vi "postPubDataUE.vi"(6 "newValue (T)":bool=TRUE, 8 "error in (no error)":errorcluster, 9 "value":variant, 10 "pubDataSV":T1=enum."LoopTime_ms", 11 "Model in":refnum<class "Model.lvclass">) -> (0 "error out":errorcluster, 3 "Model out":refnum<class "Model.lvclass">)   [LabVIEW 2016, in "Model.lvclass"]
doc: "Updates the variable value."
uses:
  Model.lvclass
  Typedefs/PubDataSV.ctl
  Model.lvclass/Model.ctl
  PubSubDataEvent/PubSubDataEvent.lvclass/PubSubDataEvent.ctl
  Typedefs/StateValue.ctl
  Typedefs/RejectedCommand.ctl
  Typedefs/CommandValue.ctl
  ComponentTemplateCore/ComponentModel/ComponentModel/Typedefs/ComponentStateValues.ctl
  PubSubDataEvent/PubSubDataEvent.lvclass
  Typedefs/EXATypedefs.lvlib
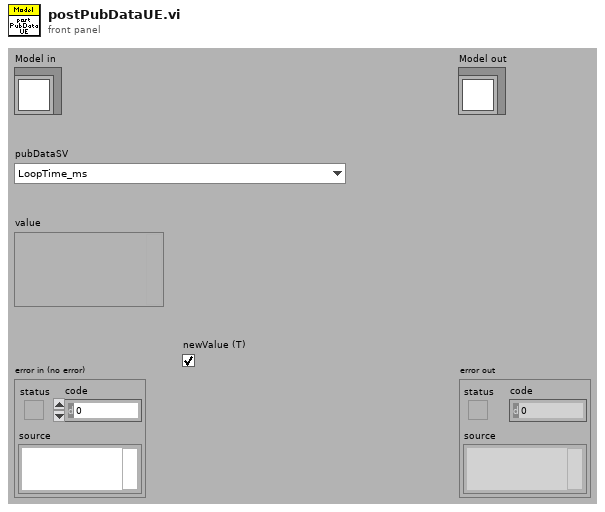
[diagram p1: front panel]
types:
  T1 = typedef "EXATypedefs.lvlib/PubDataSV.ctl" = enum16{"DetailedState", "ErrorCode", "Heartbeat", "LoopTime_ms", "LoopTimeOutOfRange", "RejectedCommand", "SummaryState", "Timestamp"}
  T2 = typedef "EXATypedefs.lvlib/PubDataEvents.ctl" = cluster{"DetailedState":refnum<user-event>, "ErrorCode":refnum<user-event>, "Heartbeat":refnum<user-event>, "LoopTime_ms":refnum<user-event>, "LoopTimeOutOfRange":refnum<user-event>, "RejectedCommand":refnum<user-event>, "SummaryState":refnum<user-event>, "Timestamp":refnum<user-event>, "AppliedSettingsMatchStart":refnum<user-event>, "SettingsApplied":refnum<user-event>, "SettingVersions":refnum<user-event>}
  T3 = typedef "EXATypedefs.lvlib/StateValue.ctl" = enum16{"DisabledState", "EnabledState", "FaultState", "OffState", "StandbyState"}
  T4 = typedef "EXATypedefs.lvlib/RejectedCommand.ctl" = cluster{"CommandValue":T5, "StateValue":T3, "Time Stamp":dbl}
  T5 = typedef "EXATypedefs.lvlib/CommandValue.ctl" = enum16{"ClearError", "Disable", "Enable", "Exit", "GoToStandby", "OnHeartbeat", "OnIncomingMessagingError", "OnInterrupt", "Start"}
  T6 = typedef "ComponentStateValues.ctl" = enum16{"Off", "Standby", "Enabled", "Disabled", "Fault"}
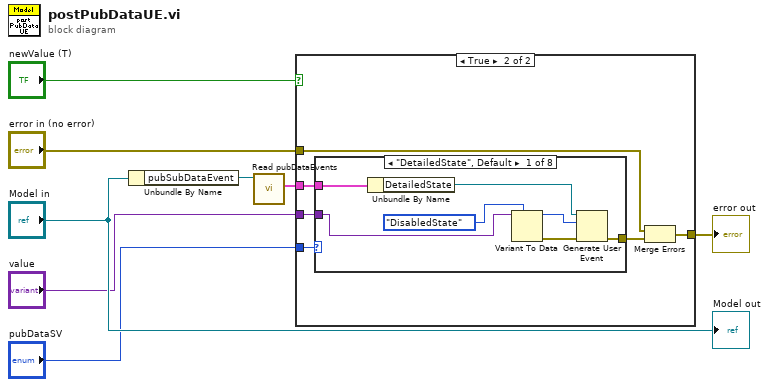
[diagram p0: block diagram]
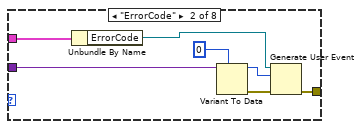
[diagram p3: hidden frame]
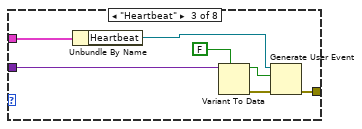
[diagram p4: hidden frame]
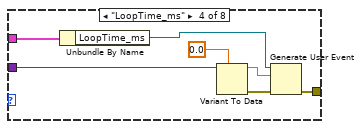
[diagram p5: hidden frame]
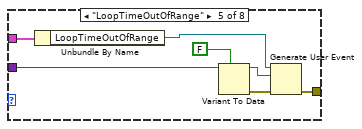
[diagram p6: hidden frame]
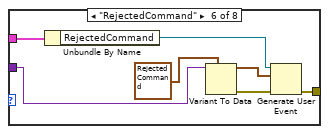
[diagram p7: hidden frame]
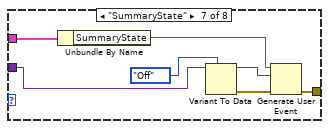
[diagram p8: hidden frame]
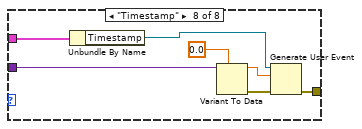
[diagram p9: hidden frame]
diagram:
  n1 = Unbundle By Name("Model in") -> ("pubSubDataEvent"=w2:refnum<class "PubSubDataEvent.lvclass">)
  n2 = call "Read pubDataEvents.vi"("PubSubDataEvent in"=w2) -> ("pubDataEvents"=w1:T2)  [unwired: 9 in, 1 out]
  n3 = case shown="True" "newValue (T)" {
    tunnel: "pubDataSV" -> [_ w12]
    tunnel: "value" -> [_ w11]
    tunnel: "error in (no error)" -> [w9 w14]
    tunnel: [w9 w15] -> w4
    tunnel: w1 -> [_ w13]
    frame False {
    }
    frame True {
      n4 = case shown="\"DetailedState\", Default" w12 {
        tunnel: w13 -> [w22 w29 w36 w43 w50 w57 w64 w71]
        tunnel: w11 -> [w20 w27 w34 w41 w48 w55 w62 w69]
        tunnel: [w19 w26 w33 w40 w47 w54 w61 w68] -> w10
        frame "DetailedState", Default {
          n5 = Unbundle By Name(w22) -> ("DetailedState"=w21:refnum<user-event>)
          n6 = Variant To Data(type=StateValue."DisabledState" ("event data"), Variant=w20) -> (data=w17:T3, error out=w16:errorcluster)  [unwired: 1 in]
          n7 = Generate User Event(user event=w21, event data cluster=w17, error in=w16) -> (error out=w19:errorcluster)  [unwired: 1 in, 1 out]
        }
        frame "ErrorCode" {
          n8 = Unbundle By Name(w29) -> ("ErrorCode"=w28:refnum<user-event>)
          n9 = Variant To Data(type=0 ("event data"), Variant=w27) -> (data=w23:i32, error out=w25:errorcluster)  [unwired: 1 in]
          n10 = Generate User Event(user event=w28, event data cluster=w23, error in=w25) -> (error out=w26:errorcluster)  [unwired: 1 in, 1 out]
        }
        frame "Heartbeat" {
          n11 = Unbundle By Name(w36) -> ("Heartbeat"=w35:refnum<user-event>)
          n12 = Variant To Data(type=FALSE ("event data"), Variant=w34) -> (data=w30:bool, error out=w32:errorcluster)  [unwired: 1 in]
          n13 = Generate User Event(user event=w35, event data cluster=w30, error in=w32) -> (error out=w33:errorcluster)  [unwired: 1 in, 1 out]
        }
        frame "LoopTime_ms" {
          n14 = Unbundle By Name(w43) -> ("LoopTime_ms"=w42:refnum<user-event>)
          n15 = Variant To Data(type=0.0 ("event data"), Variant=w41) -> (data=w37:dbl, error out=w39:errorcluster)  [unwired: 1 in]
          n16 = Generate User Event(user event=w42, event data cluster=w37, error in=w39) -> (error out=w40:errorcluster)  [unwired: 1 in, 1 out]
        }
        frame "LoopTimeOutOfRange" {
          n17 = Unbundle By Name(w50) -> ("LoopTimeOutOfRange"=w49:refnum<user-event>)
          n18 = Variant To Data(type=FALSE ("event data"), Variant=w48) -> (data=w44:bool, error out=w46:errorcluster)  [unwired: 1 in]
          n19 = Generate User Event(user event=w49, event data cluster=w44, error in=w46) -> (error out=w47:errorcluster)  [unwired: 1 in, 1 out]
        }
        frame "RejectedCommand" {
          n20 = Unbundle By Name(w57) -> ("RejectedCommand"=w56:refnum<user-event>)
          n21 = Variant To Data(type=T4 {"CommandValue"=enum."ClearError", "StateValue"=enum."DisabledState", "Time Stamp"=0.0} ("event data"), Variant=w55) -> (data=w51:T4, error out=w53:errorcluster)  [unwired: 1 in]
          n22 = Generate User Event(user event=w56, event data cluster=w51, error in=w53) -> (error out=w54:errorcluster)  [unwired: 1 in, 1 out]
        }
        frame "SummaryState" {
          n23 = Unbundle By Name(w64) -> ("SummaryState"=w63:refnum<user-event>)
          n24 = Variant To Data(type=ComponentStateValues."Off" ("event data"), Variant=w62) -> (data=w58:T6, error out=w60:errorcluster)  [unwired: 1 in]
          n25 = Generate User Event(user event=w63, event data cluster=w58, error in=w60) -> (error out=w61:errorcluster)  [unwired: 1 in, 1 out]
        }
        frame "Timestamp" {
          n26 = Unbundle By Name(w71) -> ("Timestamp"=w70:refnum<user-event>)
          n27 = Variant To Data(type=0.0 ("event data"), Variant=w69) -> (data=w65:dbl, error out=w67:errorcluster)  [unwired: 1 in]
          n28 = Generate User Event(user event=w70, event data cluster=w65, error in=w67) -> (error out=w68:errorcluster)  [unwired: 1 in, 1 out]
        }
      }
      n29 = Merge Errors(w14, w10) -> (w15:errorcluster)
    }
  }
  "error out" <- w4
  "Model out" <- "Model in"
